vi "Robot Lift Speed Selection.vi"(11 "upper limit in":dbl) -> (3 "upper limit out":dbl)   [LabVIEW 2017]
uses:
  <vilib>/Rock Robotics/Network Tables/NT Read Number.vi
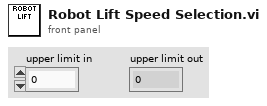
[diagram p1: front panel]
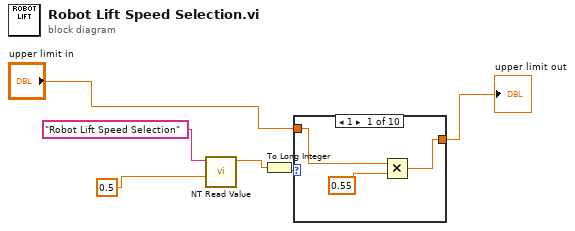
[diagram p0: block diagram]
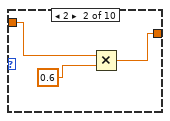
[diagram p2: hidden frame]
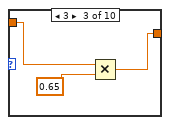
[diagram p3: hidden frame]
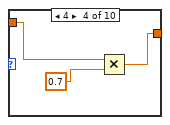
[diagram p4: hidden frame]
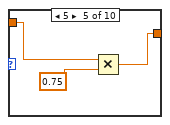
[diagram p5: hidden frame]
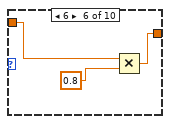
[diagram p6: hidden frame]
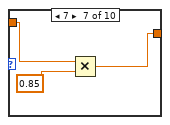
[diagram p7: hidden frame]
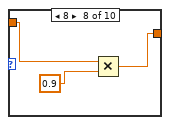
[diagram p8: hidden frame]
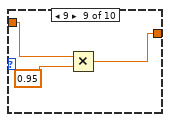
[diagram p9: hidden frame]
diagram:
  n1 = call-poly <vilib>:"NT Read Value.vi"("Default Value"=0.5, "Name"="Robot Lift Speed Selection") -> ("Numeric"=w2:dbl)  [unwired: 8 in, 1 out]
  n2 = To Long Integer(number=w2) -> (32bit integer=w1:i32)
  n3 = case shown="1" w1 {
    tunnel: "upper limit in" -> [w8 w11 w14 w17 w20 w23 w26 w29 w32 w34]
    tunnel: [w7 w10 w13 w16 w19 w22 w25 w28 w31 w34] -> w6
    frame 1 {
      n4 = Multiply(x=w8, y=0.55) -> (x*y=w7:dbl)
    }
    frame 2 {
      n5 = Multiply(x=w11, y=0.6) -> (x*y=w10:dbl)
    }
    frame 3 {
      n6 = Multiply(x=w14, y=0.65) -> (x*y=w13:dbl)
    }
    frame 4 {
      n7 = Multiply(x=w17, y=0.7) -> (x*y=w16:dbl)
    }
    frame 5 {
      n8 = Multiply(x=w20, y=0.75) -> (x*y=w19:dbl)
    }
    frame 6 {
      n9 = Multiply(x=w23, y=0.8) -> (x*y=w22:dbl)
    }
    frame 7 {
      n10 = Multiply(x=w26, y=0.85) -> (x*y=w25:dbl)
    }
    frame 8 {
      n11 = Multiply(x=w29, y=0.9) -> (x*y=w28:dbl)
    }
    frame 9 {
      n12 = Multiply(x=w32, y=0.95) -> (x*y=w31:dbl)
    }
    frame 10, Default {
    }
  }
  "upper limit out" <- w6
